vi "电导率_所有参数读取.vi"(8 "error in (no error)":errorcluster caption="错误输入（无错误）", 11 "MB session in":refnum<class "MB_Master.lvclass">) -> (0 "error out":errorcluster caption="错误输出", 2 "输出值":T1 {"电极型号标志" items=["NULL", "pH", "Cond", "DO", "Turb"]; "电极状态标志" items=["OK"]}, 3 "MB session out":refnum<class "MB_Master.lvclass">)   [LabVIEW 2022 SP3, in "斯坦道多参数.lvlib"]
uses:
  <vilib>/Plasmionique/MB Master/MB_Master/MB_Master.lvclass
  <vilib>/Plasmionique/MB Master/MB Master.lvlib
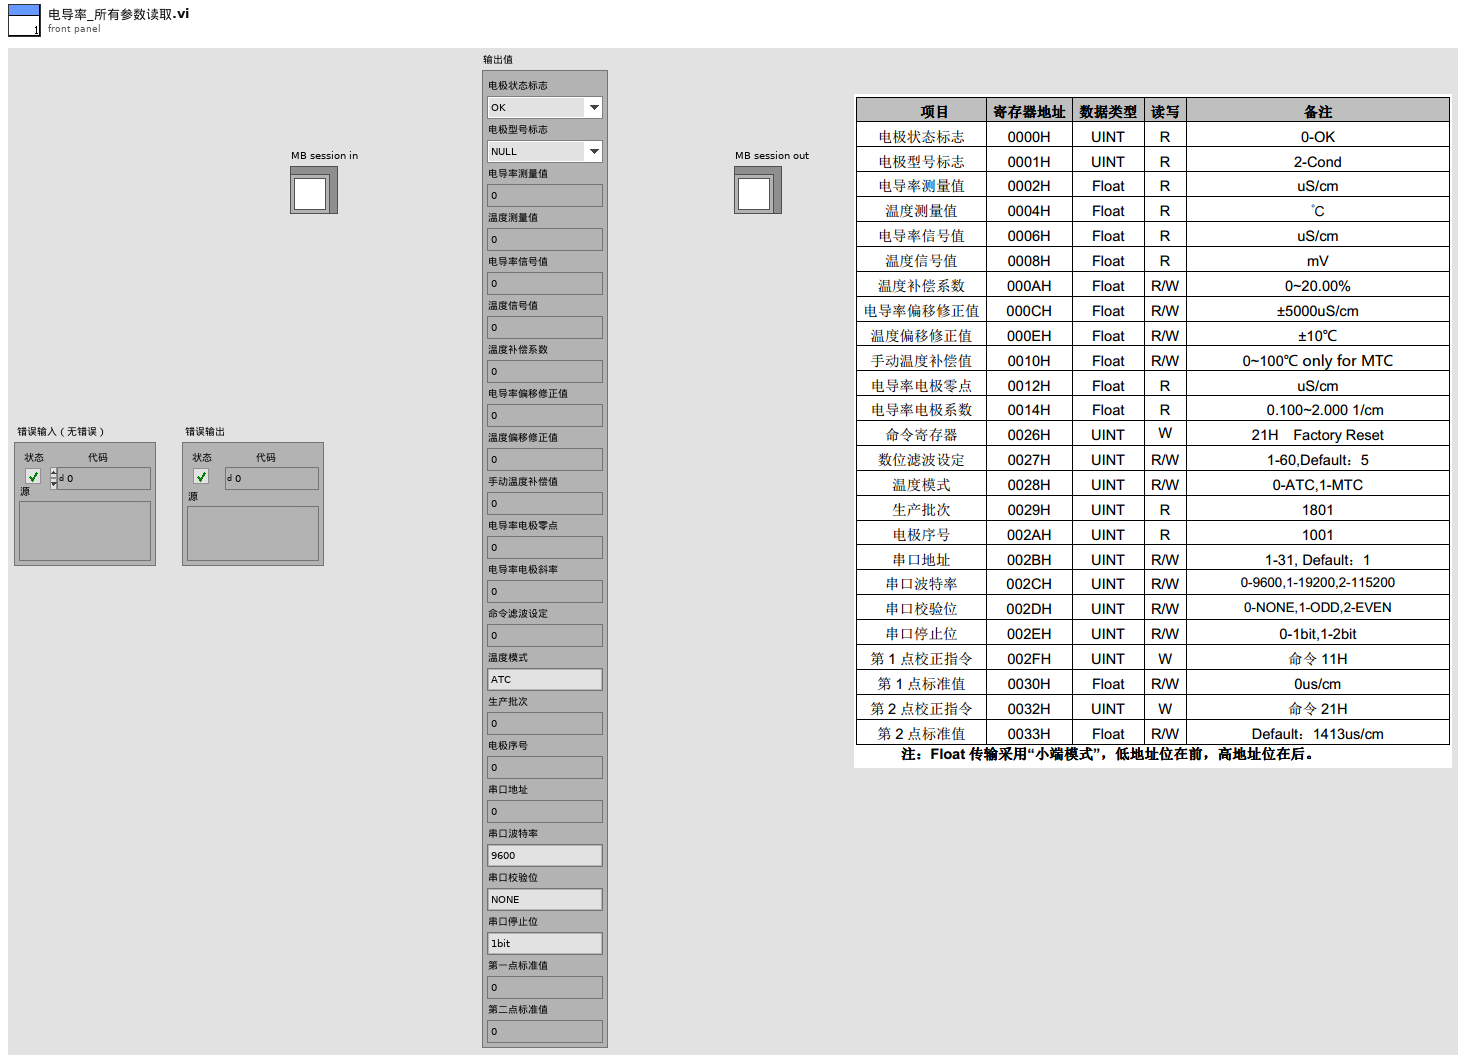
[diagram p1: front panel]
types:
  T1 = cluster{"电极状态标志":u16, "电极型号标志":u16, "电导率测量值":sgl, "温度测量值":sgl, "电导率信号值":sgl, "温度信号值":sgl, "温度补偿系数":sgl, "电导率偏移修正值":sgl, "温度偏移修正值":sgl, "手动温度补偿值":sgl, "电导率电极零点":sgl, "电导率电极斜率":sgl, "命令滤波设定":u16, "温度模式":enum16{"ATC", "MTC"}, "生产批次":u16, "电极序号":u16, "串口地址":u16, "串口波特率":enum16{"9600", "19200", "115200"}, "串口校验位":enum16{"NONE", "ODD", "EVEN"}, "串口停止位":enum16{"1bit", "2bit"}, "第一点标准值":sgl, "第二点标准值":sgl}
  T2 = cluster{u16, u16, "数值":sgl, "数值":sgl, "数值":sgl, "数值":sgl, "数值":sgl, "数值":sgl, "数值":sgl, "数值":sgl, "数值":sgl, "数值":sgl, u16, u16, u16, u16, u16, u16, u16, u16, "数值":sgl, "数值":sgl}
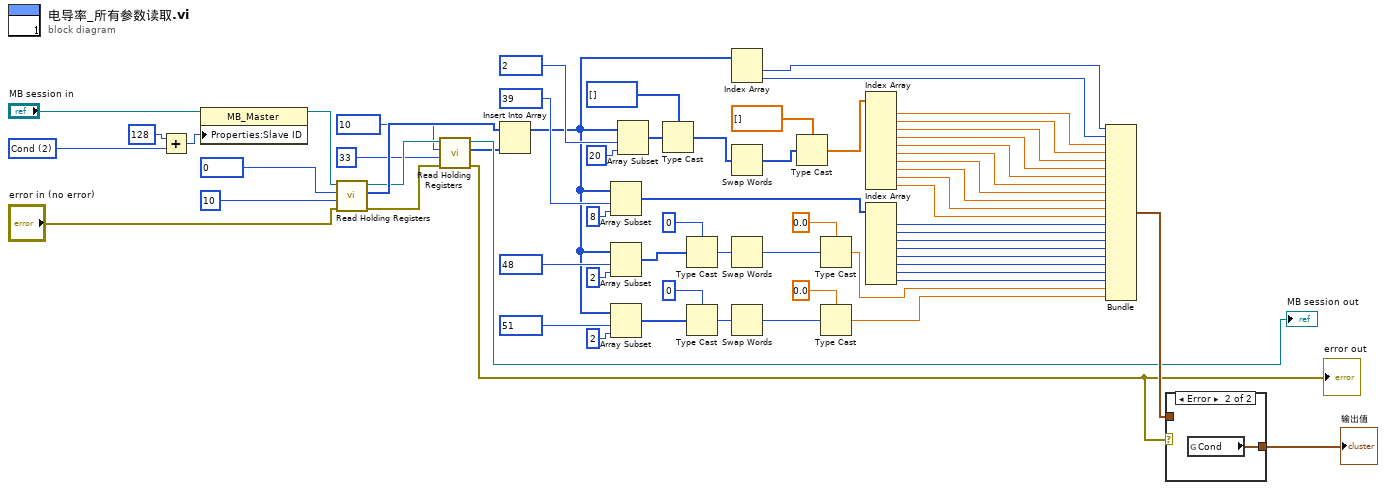
[diagram p0: block diagram]
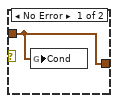
[diagram p2: hidden frame]
diagram:
  w66 = u16 2 items=["NULL", "pH", "Cond", "DO", "Turb"] ("数值")
  n1 = Add(x=u16 128, y=w66) -> (x+y=w65:u16)
  n2 = property class="MB_Master"(reference="MB session in", "Properties:Slave ID"=w65) -> (reference out=w19:refnum<class "MB_Master.lvclass">)  [unwired: 1 in, 1 out]
  n3 = call <vilib>:"Read Holding Registers.vi"("error in (no error)"="error in (no error)", "quantity"=u16 10, "starting address"=u16 0, "MB session in"=w19) -> ("error out"=w6:errorcluster, "Registers"=w33:u16[], "MB session out"=w8:refnum<class "MB_Master.lvclass">)  [unwired: 5 in]
  n4 = call <vilib>:"Read Holding Registers.vi"("error in (no error)"=w6, "quantity"=u16 33, "starting address"=u16 10, "MB session in"=w8) -> ("error out"=w5:errorcluster, "Registers"=w1:u16[], "MB session out"=→"MB session out":refnum<class "MB_Master.lvclass">)  [unwired: 5 in]
  "error out" <- w5
  n5 = Insert Into Array(array=w33, new element=w1) -> (w2:u16[])  [unwired: 1 in]
  n6 = Array Subset(array=w2, index=u16 39 ("starting address"), length=8 ("长度")) -> (w46:u16[])
  n7 = Array Subset(array=w2, index=u16 48 ("starting address"), length=2 ("长度")) -> (w28:u16[])
  n8 = Array Subset(array=w2, index=u16 51 ("starting address"), length=2 ("长度")) -> (w23:u16[])
  n9 = Array Subset(array=w2, index=u16 2 ("starting address"), length=20 ("长度")) -> (w54:u16[])
  n10 = Type Cast(type=u32[] [] ("数组 2"), x=w54) -> (*(type *) &x=w56:u32[])
  n11 = Type Cast(type=u32 0 ("数值"), x=w28) -> (*(type *) &x=w31:u32)
  n12 = Type Cast(type=u32 0 ("数值"), x=w23) -> (*(type *) &x=w25:u32)
  n13 = Index Array(array=w2) -> (element #1=w61:u16, element #2=w60:u16)  [unwired: 2 in]
  n14 = Swap Words(1:w56) -> (0:w58:u32[])
  n15 = Swap Words(1:w31) -> (0:w32:u32)
  n16 = Swap Words(1:w25) -> (0:w24:u32)
  n17 = Type Cast(type=sgl[] [] ("数组 2"), x=w58) -> (*(type *) &x=w53:sgl[])
  n18 = Type Cast(type=sgl 0.0 ("数值"), x=w32) -> (*(type *) &x=w22:sgl)
  n19 = Type Cast(type=sgl 0.0 ("数值"), x=w24) -> (*(type *) &x=w21:sgl)
  n20 = Index Array(array=w53) -> (element #1=w10:sgl, element #2=w52:sgl, element #3=w51:sgl, element #4=w50:sgl, element #5=w18:sgl, element #6=w17:sgl, element #7=w16:sgl, element #8=w15:sgl, element #9=w14:sgl, element #10=w13:sgl)  [unwired: 10 in]
  n21 = Index Array(array=w46) -> (element #1=w45:u16, element #2=w44:u16, element #3=w43:u16, element #4=w42:u16, element #5=w41:u16, element #6=w40:u16, element #7=w39:u16, element #8=w38:u16)  [unwired: 8 in]
  n22 = Bundle(w61, w60, "数值"=w10, "数值"=w52, "数值"=w51, "数值"=w50, "数值"=w18, "数值"=w17, "数值"=w16, "数值"=w15, "数值"=w14, "数值"=w13, w45, w44, w43, w42, w41, w40, w39, w38, "数值"=w22, "数值"=w21) -> (w12:T2)  [unwired: 1 in]
  n23 = case shown="Error" w5 {
    tunnel: w12 -> [w67 _]
    tunnel: [w67 w68] -> w9
    frame No Error {
      n24 = global write "国弘过程全局变量.vi" "Cond"(w67) -> ()
    }
    frame Error {
      n25 = global read "国弘过程全局变量.vi" "Cond"() -> (w68:T1)
    }
  }
  "输出值" <- w9
